vi "XYsave_txt.vi"(1 "Correct deflection":bool, 2 "Cluster":T1, 3 "error in (no error)":errorcluster, 4 "datalog path (use dialog)":path) -> (0 "error out":errorcluster)   [LabVIEW 2013]
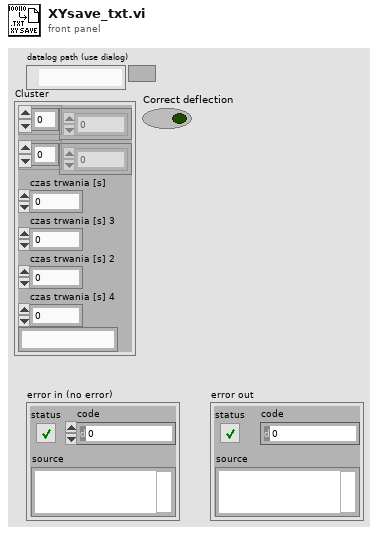
[diagram p1: front panel]
types:
  T1 = cluster{dbl[], dbl[], "czas trwania [s]":dbl, "czas trwania [s] 3":dbl, "czas trwania [s] 2":dbl, "czas trwania [s] 4":dbl, string}
  T2 = enum16{"open", "replace", "create", "open or create", "replace or create", "replace or create with confirmation"}
  T3 = typedef "NI_Matrix.lvlib/RealMatrix.ctl" = dbl[][]
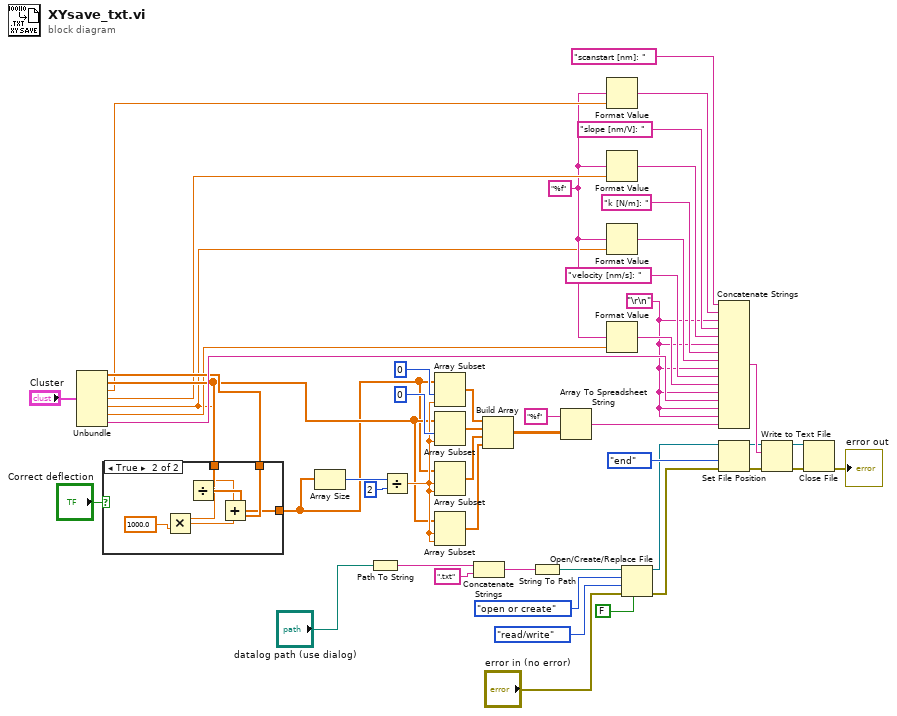
[diagram p0: block diagram]
diagram:
  w3 = "%f" ("format string")
  w12 = "\r\n"
  n1 = Unbundle("Cluster") -> (w10:dbl[], w9:dbl[], "czas trwania [s]"=w7:dbl, "czas trwania [s] 3"=w4:dbl, "czas trwania [s] 2"=w2:dbl, "czas trwania [s] 4"=w5:dbl, w13:string)
  n2 = case shown="True" "Correct deflection" {
    tunnel: w10 -> [w51 w57]
    tunnel: w9 -> [_ w56]
    tunnel: [w51 w55] -> w8
    tunnel: w2 -> [_ w54]
    frame False {
    }
    frame True {
      n3 = Multiply(x=w54, y=1000.0) -> (x*y=w52:dbl)
      n4 = Divide(x=w56, y=w52) -> (x/y=w58:dbl[])
      n5 = Add(x=w58, y=w57) -> (x+y=w55:dbl[])
    }
  }
  n6 = Array Size(array=w8) -> (size(s)=w19:i32)
  n7 = Path To String(path="datalog path (use dialog)") -> (string=w44:string)
  n8 = Divide(x=w19, y=2) -> (x/y=w17:dbl)
  n9 = Array Subset(array=w8, index=0, length=w17) -> (w21:dbl[])
  n10 = Array Subset(array=w9, index=0, length=w17) -> (w15:dbl[])
  n11 = Array Subset(array=w8, index=w17, length=w17) -> (w16:dbl[])
  n12 = Array Subset(array=w9, index=w17, length=w17) -> (w20:dbl[])
  n13 = Concatenate Strings(w44, ".txt") -> (w45:string)
  n14 = Build Array(w21, w15, w16, w20) -> (w32:T3)
  n15 = String To Path(string=w45) -> (path=w47:path)
  n16 = Array To Spreadsheet String(array=w32, 3:"%f" ("format string")) -> (spreadsheet string=w11:string)  [unwired: 1 in]
  n17 = Format Value(format string=w3, value (0)=w7) -> (output string=w6:string)  [unwired: 1 in]
  n18 = Format Value(format string=w3, value (0)=w4) -> (output string=w39:string)  [unwired: 1 in]
  n19 = Format Value(format string=w3, value (0)=w2) -> (output string=w38:string)  [unwired: 1 in]
  n20 = Format Value(format string=w3, value (0)=w5) -> (output string=w37:string)  [unwired: 1 in]
  n21 = Open/Create/Replace File(file path (use dialog)=w47, error in="error in (no error)", operation (0:open)=T2."open or create", access (0:read/write)=enum16{"read/write", "read-only", "write-only"}."read/write", disable buffering (F)=FALSE) -> (refnum out=w24:refnum<file>, error out=w25:errorcluster)  [unwired: 1 in, 1 out]
  n22 = Concatenate Strings("scanstart [nm]: ", w6, w12, "slope [nm/V]: ", w39, w12, "k [N/m]: ", w38, w12, "velocity [nm/s]: ", w37, w12, w13, w12, w12, w11) -> (w28:string)
  n23 = Set File Position(refnum=w24, from (0:start)=enum16{"start", "end", "current"}."end", error in=w25) -> (refnum out=w26:refnum<file>, error out=w27:errorcluster)  [unwired: 1 in]
  n24 = Write to Text File(file (use dialog)=w26, text=w28, error in=w27) -> (refnum out=w29:refnum<file>, error out=w30:errorcluster)  [unwired: 1 in, 1 out]
  n25 = Close File(refnum=w29, error in=w30) -> (error out=→"error out":errorcluster)  [unwired: 1 out]
